vi "VI Tree.vi"   [LabVIEW 2017, in "Lake Shore 336.lvlib"]
doc: "This is the instrument driver for the Lake Shore Model 336 Temperature Controller. The VI Tree displays all the user-callable VIs of the instrument driver in an organized table."
uses:
  Lake Shore 336.lvlib
  Data/Sensor Data (Multiple Readings).vi
panel:
  # "(c) 2009 Lake Shore Cryotronics Inc.  ALL RIGHTS RESERVED."
  # "SEE DIAGRAM\nFOR VI TREE."
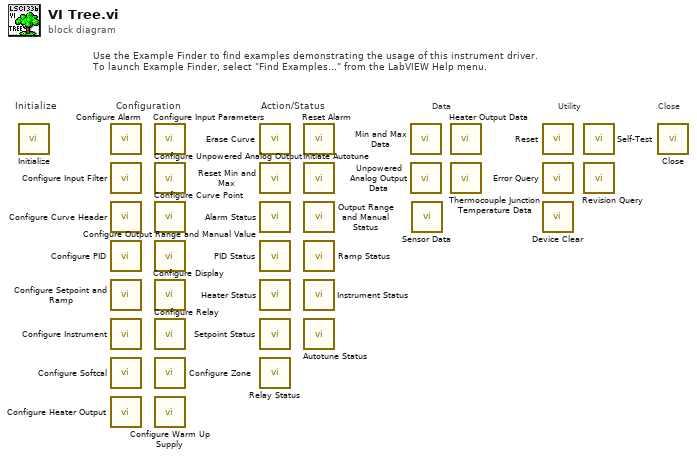
[diagram p0: block diagram]
diagram:
  # "Configuration"
  # "Utility"
  # "Data"
  # "Action/Status"
  # "Close"
  # "Initialize"
  # "Use the Example Finder to find examples demonstrating the usage of this instrument driver.\nTo launch Example Finder, select \"Find Examples...\" from the LabVIEW Help menu."
  n1 = call "Initialize.vi"() -> ()  [unwired: 10 in, 2 out]
  n2 = call "Configure Alarm.vi"() -> ()  [unwired: 14 in, 2 out]
  n3 = call "Configure Input Filter.vi"() -> ()  [unwired: 14 in, 2 out]
  n4 = call "Configure Curve Header.vi"() -> ()  [unwired: 14 in, 2 out]
  n5 = call "Configure PID.vi"() -> ()  [unwired: 14 in, 2 out]
  n6 = call "Configure Setpoint and Ramp.vi"() -> ()  [unwired: 14 in, 2 out]
  n7 = call "Configure Instrument.vi"() -> ()  [unwired: 14 in, 2 out]
  n8 = call "Configure Softcal.vi"() -> ()  [unwired: 14 in, 2 out]
  n9 = call "Configure Heater Output.vi"() -> ()  [unwired: 14 in, 2 out]
  n10 = call "Configure Input Parameters.vi"() -> ()  [unwired: 14 in, 2 out]
  n11 = call "Configure Unpowered Analog Output.vi"() -> ()  [unwired: 14 in, 2 out]
  n12 = call "Configure Curve Point.vi"() -> ()  [unwired: 14 in, 2 out]
  n13 = call "Configure Output Range and Manual Value.vi"() -> ()  [unwired: 14 in, 2 out]
  n14 = call "Configure Display.vi"() -> ()  [unwired: 14 in, 2 out]
  n15 = call "Configure Relay.vi"() -> ()  [unwired: 14 in, 2 out]
  n16 = call "Configure Zone.vi"() -> ()  [unwired: 14 in, 2 out]
  n17 = call "Configure Warm Up Supply.vi"() -> ()  [unwired: 14 in, 2 out]
  n18 = call "Erase Curve.vi"() -> ()  [unwired: 10 in, 2 out]
  n19 = call "Reset Min and Max.vi"() -> ()  [unwired: 10 in, 2 out]
  n20 = call "Alarm Status.vi"() -> ()  [unwired: 8 in, 4 out]
  n21 = call "PID Status.vi"() -> ()  [unwired: 7 in, 5 out]
  n22 = call "Heater Status.vi"() -> ()  [unwired: 9 in, 3 out]
  n23 = call "Setpoint Status.vi"() -> ()  [unwired: 9 in, 3 out]
  n24 = call "Relay Status.vi"() -> ()  [unwired: 9 in, 3 out]
  n25 = call "Reset Alarm.vi"() -> ()  [unwired: 10 in, 2 out]
  n26 = call "Initiate Autotune.vi"() -> ()  [unwired: 14 in, 2 out]
  n27 = call "Output Range and Manual Status.vi"() -> ()  [unwired: 8 in, 4 out]
  n28 = call "Ramp Status.vi"() -> ()  [unwired: 7 in, 5 out]
  n29 = call "Instrument Status.vi"() -> ()  [unwired: 7 in, 5 out]
  n30 = call "Autotune Status.vi"() -> ()  [unwired: 6 in, 6 out]
  n31 = call "Min and Max Data.vi"() -> ()  [unwired: 8 in, 4 out]
  n32 = call "Unpowered Analog Output Data.vi"() -> ()  [unwired: 9 in, 3 out]
  n33 = call-poly "Sensor Data.vi"() -> ()  [unwired: 9 in, 3 out]
  n34 = call "Heater Output Data.vi"() -> ()  [unwired: 9 in, 3 out]
  n35 = call "Thermocouple Junction Temperature Data.vi"() -> ()  [unwired: 9 in, 3 out]
  n36 = call "Reset.vi"() -> ()  [unwired: 10 in, 2 out]
  n37 = call "Error Query.vi"() -> ()  [unwired: 9 in, 3 out]
  n38 = call "Device Clear.vi"() -> ()  [unwired: 10 in, 2 out]
  n39 = call "Self-Test.vi"() -> ()  [unwired: 8 in, 4 out]
  n40 = call "Revision Query.vi"() -> ()  [unwired: 5 in, 7 out]
  n41 = call "Close.vi"() -> ()  [unwired: 11 in, 1 out]
